vi "Detected DPIs.vi"() -> (0 "error out":errorcluster, 2 "DPI resources":string[](array[string]))   [LabVIEW 2021]
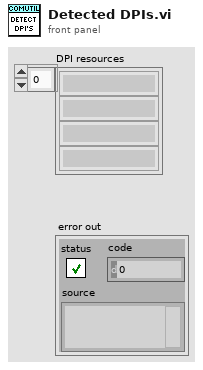
[diagram p1: front panel]
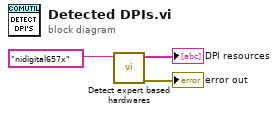
[diagram p0: block diagram]
diagram:
  n1 = call "Detect expert based hardwares.vi"("Expert name"="nidigital657x") -> ("error out"=→"error out":errorcluster, "Alias names"=→"DPI resources":string[])  [unwired: 8 in, 1 out]
